vi "One-ENC.vi"(7 "Reset":bool, 8 "Error In":errorcluster) -> (0 "Error Out":errorcluster, 3 "Counter Value":dbl)   [LabVIEW 2019]
uses:
  <vilib>/Utility/error.llb/Error Cluster From Error Code.vi
  <vilib>/myRIO/Common/Instrument Driver Framework/myRIO v1.0/Encoder/vis/myRIO v1.0 Read Encoder.vi
  <vilib>/myRIO/Instrument Drivers/Onboard IO/Encoder/Encoder.lvlib
panel:
  out "Waveform Chart":dbl(graph)
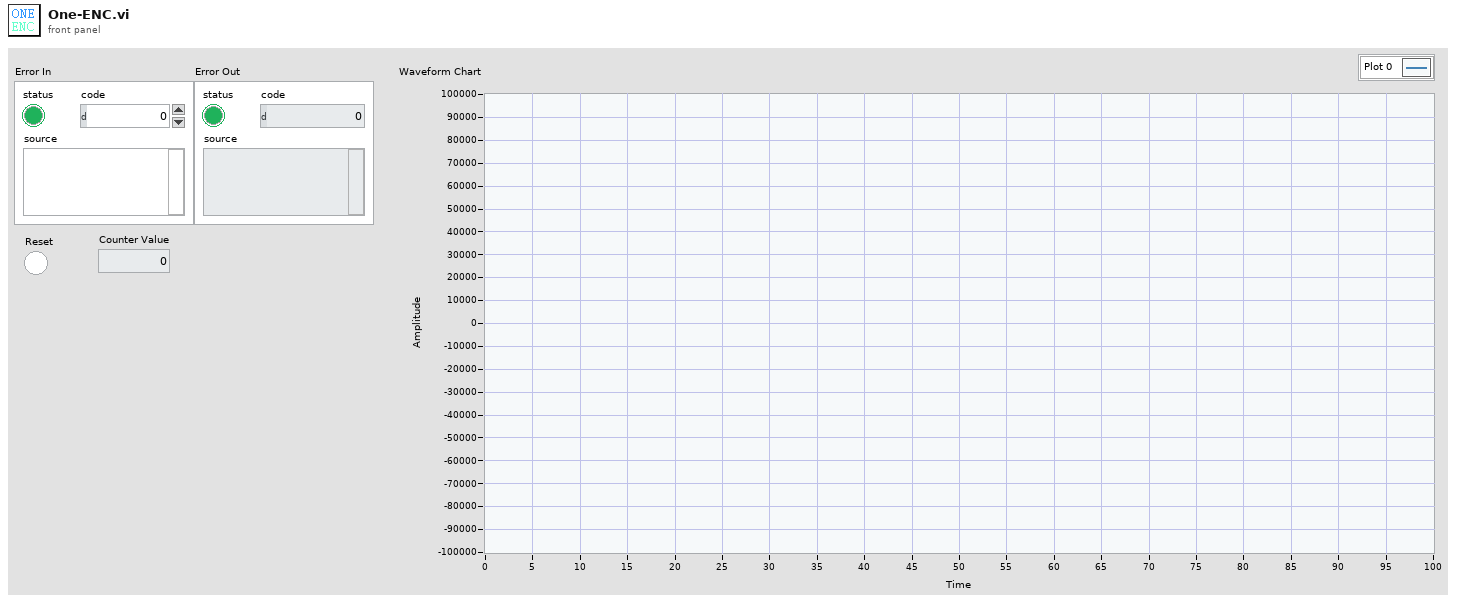
[diagram p1: front panel]
types:
  T1 = typedef "Encoder.lvlib/Encoder Reference.ctl" = cluster{"myRIO Reference":T2, "Encoder Channels Enum":T6}
  T2 = typedef "myRIO Generic Hardware Reference.ctl" = cluster{"myRIO Model":T3, "myRIO Hardware Reference":T4}
  T3 = typedef "Hardware Version Enum.ctl" = enum16{"Unknown", "myRIO-1900", "myRIO-1950", "roboRIO", "NI ELVIS RIO CM", "ELVIS III"}
  T4 = typedef "myRIO v1.0 Reference.ctl" = cluster{"Generic FPGA Reference":T5, "Allow multiple opens":bool}
  T5 = typedef "Generic FPGA Reference.ctl" = refnum<k20>
  T6 = typedef "Encoder Channels Enum.ctl" = enum16{"Not Connected", "C/ENC0", "C/ENC1", "A/ENC", "A/ENC0", "A/ENC1", "A/ENC2", "A/ENC3", "A/ENC4", "A/ENC5", "A/ENC6", "A/ENC7", "A/ENC8", "A/ENC9", "B/ENC", "B/ENC0", "B/ENC1", "B/ENC2", "B/ENC3", "B/ENC4", "B/ENC5", "B/ENC6", "B/ENC7", "B/ENC8", "B/ENC9", "DIO/ENC0", "DIO/ENC1", "DIO/ENC2", "DIO/ENC3", "DIO/ENC4"}
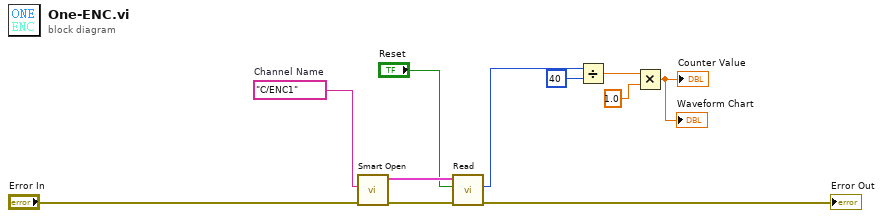
[diagram p0: block diagram]
diagram:
  w9 = tag "C/ENC1"  # Channel Name
  n1 = call <vilib>:"Smart Open.vi"("error in (no error)"="Error In", "Channel Name"=w9) -> ("error out"=w7:errorcluster, "Encoder Ref Out"=w8:T1)  [unwired: 8 in]
  n2 = call <vilib>:"Read.vi"("error in (no error)"=w7, "Reset Counter"="Reset", "Encoder Ref In"=w8) -> ("error out"=→"Error Out":errorcluster, "Counter Value"=w6:i32)  [unwired: 4 in, 3 out]
  n3 = Divide(x=w6, y=40) -> (x/y=w3:dbl)
  n4 = Multiply(x=w3, y=1.0) -> (x*y=→"Counter Value" →"Waveform Chart":dbl)
